vi "form voltage alarm string.old.vi"(0 "Xmon":dbl[][](array[numeric]), 1 "Xset":dbl[][](array[numeric]), 2 "Timestamps":dbl[][](array[numeric]), 3 "Alarm Tolerance (frac)":dbl=0.2 format="%#_13g", 4 "Warning Tolerance (frac)":dbl=0.1 format="%#_13g", 5 "error in":errorcluster, 6 "Alarm:T Warning:F":bool, 8 "Current:T Voltage:F":bool, 12 "Start index":i32) -> (14 "Error Status String":string, 15 "All channels in error":string, 17 "Error Array":string[][](array[string]), 19 "Error Out":errorcluster)   [LabVIEW 2015]
uses:
  CAEN globals.vi
  <userlib>/_OpenG.lib/array/array.llb/Search 1D Array (Boolean)__ogtk.vi
  <userlib>/_OpenG.lib/array/array.llb/Index 1D Array Elements (I32)__ogtk.vi
  <userlib>/_OpenG.lib/array/array.llb/Index 1D Array Elements (Boolean)__ogtk.vi
  <userlib>/_OpenG.lib/array/array.llb/Index 1D Array Elements (String)__ogtk.vi
  <userlib>/_OpenG.lib/array/array.llb/Index 1D Array Elements (DBL)__ogtk.vi
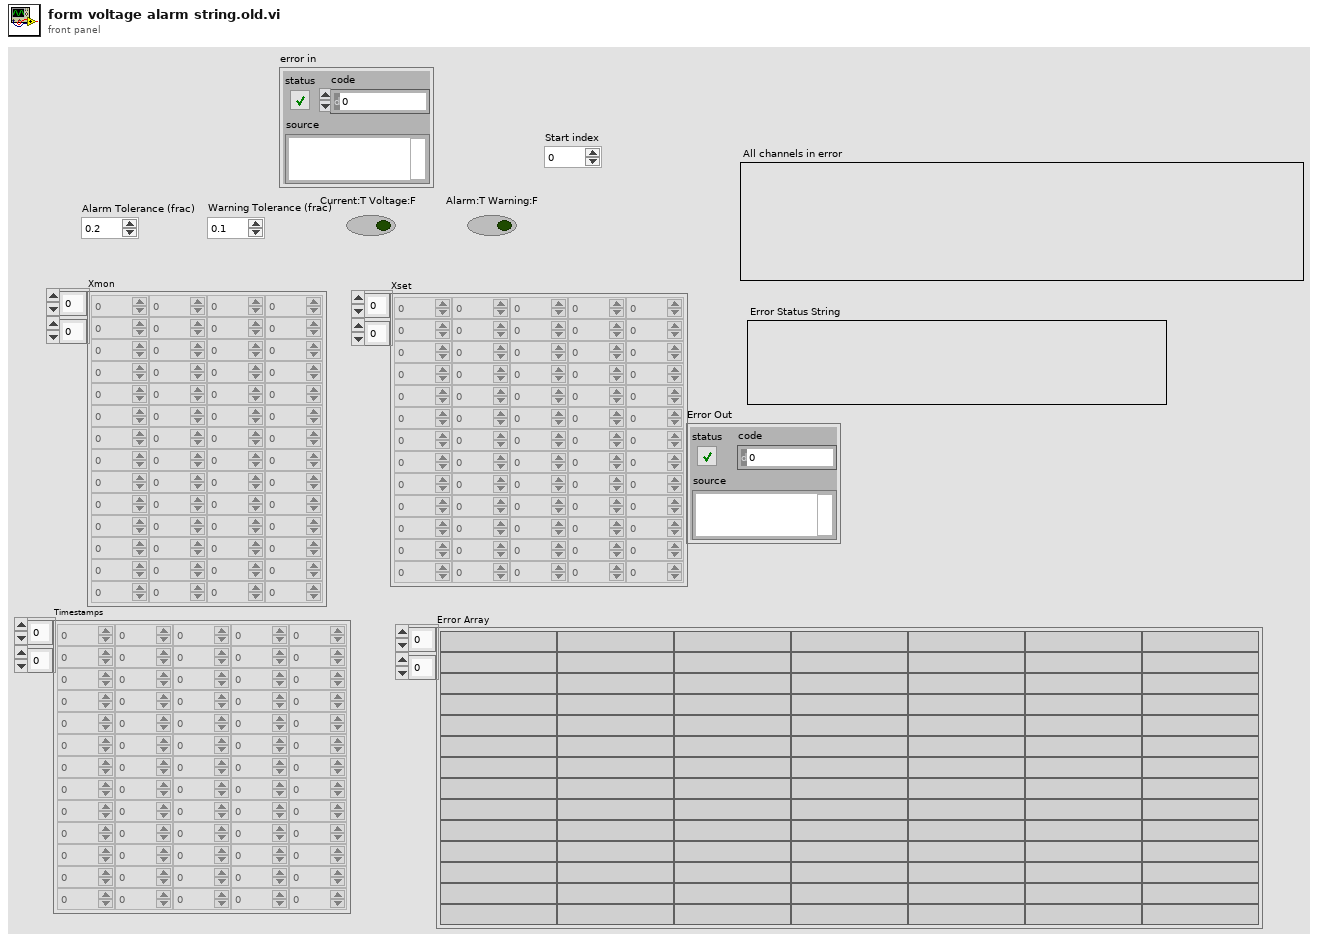
[diagram p1: front panel]
types:
  T1 = cluster{"Slot num":i32, "Indices of Elements":i32[]}[]
  T2 = cluster{"Channel Name":string, "Crate":i32, "Card Type":string, "Card":i32, "Channel":i32, "Status Icon":picture, "Vmon (V)":dbl, "Vset (V)":dbl, "Imon (A)":dbl, "Iset (A)":dbl, "Timestamp":string, "ON/OFF":bool, "Status":string, "Vswmax (V)":dbl}[]
  T3 = cluster{"Channel Name":string, "Crate":i32, "Card Type":string, "Card":i32, "Channel":i32, "Status Icon":picture, "Vmon (V)":dbl, "Vset (V)":dbl, "Imon (A)":dbl, "Iset (A)":dbl, "Timestamp":string, "ON/OFF":bool, "Status":string, "Vswmax (V)":dbl}
  T4 = cluster{"Numeric":i32, "Indices of Elements":i32[]}
  T5 = cluster{"Numeric":i32, "Indices of Elements":i32[]}[]
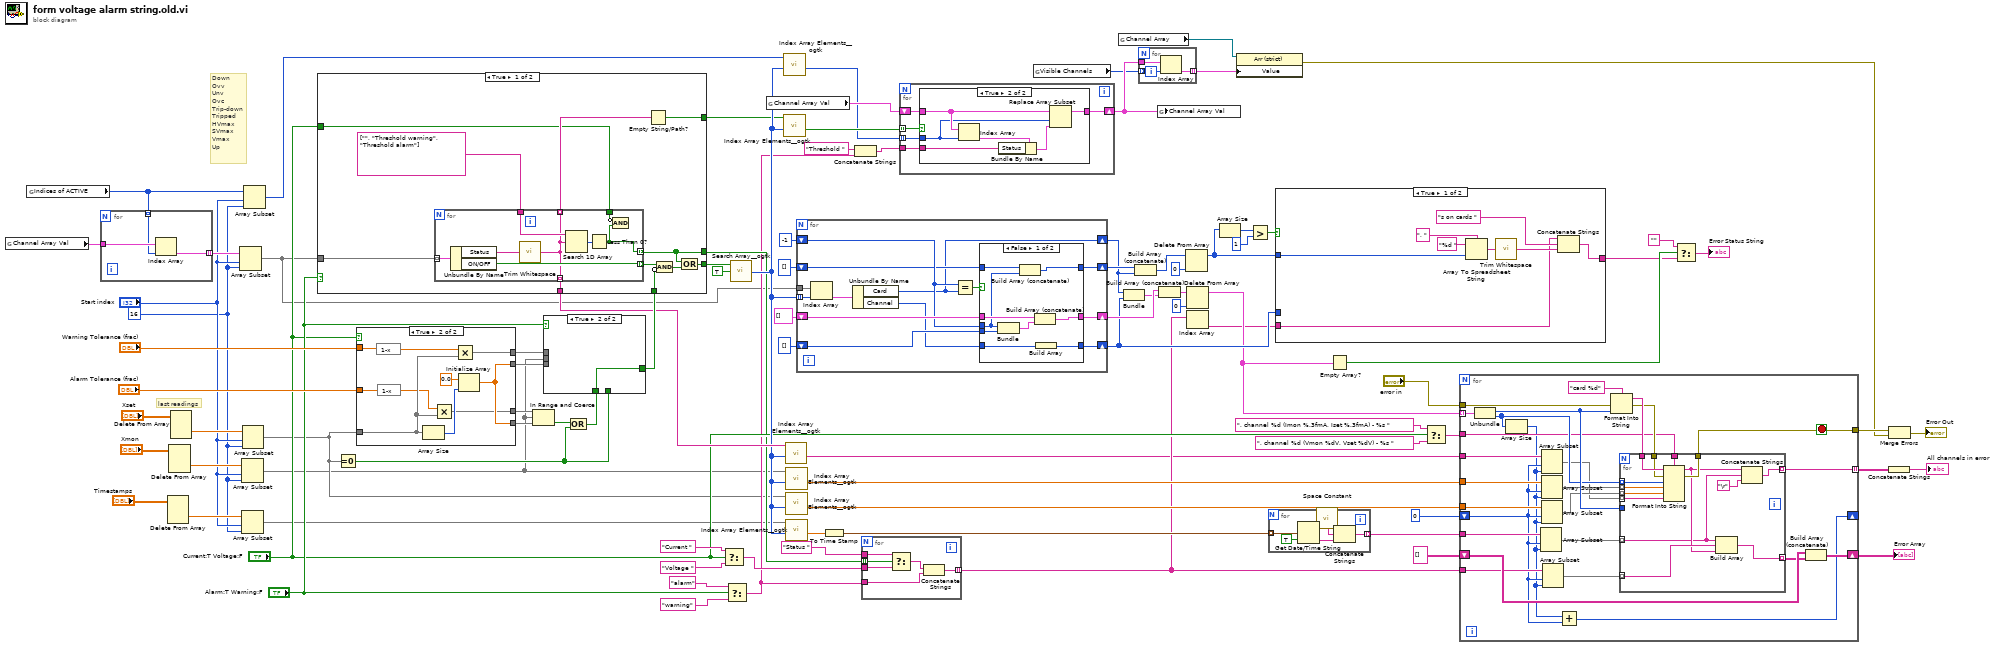
[diagram p0: block diagram]
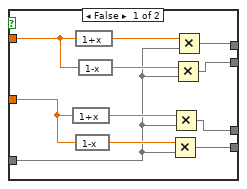
[diagram p3: hidden frame]
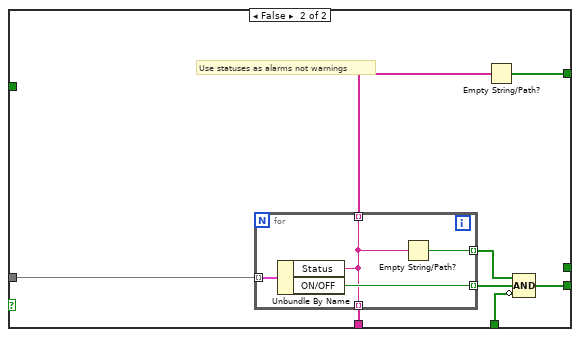
[diagram p4: hidden frame]
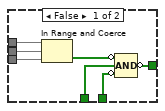
[diagram p5: hidden frame]
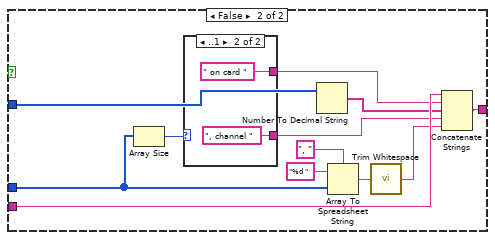
[diagram p6: hidden frame]
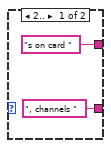
[diagram p7: hidden frame]
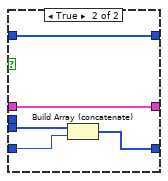
[diagram p8: hidden frame]
diagram:
  w2 = 16 ("Length")
  # "Down\nOvv\nUnv\nOvc\nTrip-down\nTripped\nHVmax\nSVmax\nVmax\nUp"
  # "last readings"
  n1 = global read "CAEN globals.vi" "Channel Array Val"() -> (w39:T2)
  n2 = global read "CAEN globals.vi" "Indices of ACTIVE"() -> (w5:i32[])
  n3 = for {
    tunnel: w39 -> [w95]
    tunnel: [w94] -> w6 mode=indexing
    tunnel: w5 -> [w93] mode=indexing
    n4 = Index Array(array=w95, index=w93) -> (element=w94:T3)
  }
  n5 = Delete From Array(array="Timestamps") -> (deleted portion=w9:dbl[])  [unwired: 3 in, 1 out]
  n6 = Delete From Array(array="Xmon") -> (deleted portion=w11:dbl[])  [unwired: 3 in, 1 out]
  n7 = Delete From Array(array="Xset") -> (deleted portion=w13:dbl[])  [unwired: 3 in, 1 out]
  n8 = Array Subset(array=w6, index="Start index", length=w2) -> (w7:T2)
  n9 = Array Subset(array=w11, index="Start index", length=w2) -> (w10:dbl[])
  n10 = Array Subset(array=w9, index="Start index", length=w2) -> (w8:dbl[])
  n11 = Array Subset(array=w13, index="Start index", length=w2) -> (w12:dbl[])
  n12 = Array Subset(array=w5, index="Start index", length=w2) -> (w4:i32[])
  n13 = Equal To 0?(x=w12) -> (x = 0?=w46:bool[])
  n14 = case shown="True" "Current:T Voltage:F" {
    tunnel: [w98 w114] -> w63
    tunnel: [w99 w109] -> w62
    tunnel: [w104 w111] -> w45
    tunnel: [w102 w114] -> w44
    tunnel: "Warning Tolerance (frac)" -> [w106 w112]
    tunnel: "Alarm Tolerance (frac)" -> [w97 w110]
    tunnel: w12 -> [w96 w113]
    frame False {
      n15 = expression code="1+x"(w97) -> (w100:dbl)
      n16 = expression code="1+x"(w106) -> (w105:dbl)
      n17 = expression code="1-x"(w97) -> (w101:dbl)
      n18 = expression code="1-x"(w106) -> (w103:dbl)
      n19 = Multiply(x=w101, y=w96) -> (x*y=w98:dbl[])
      n20 = Multiply(x=w100, y=w96) -> (x*y=w99:dbl[])
      n21 = Multiply(x=w103, y=w96) -> (x*y=w102:dbl[])
      n22 = Multiply(x=w105, y=w96) -> (x*y=w104:dbl[])
    }
    frame True {
      n23 = expression code="1-x"(w112) -> (w108:dbl)
      n24 = expression code="1-x"(w110) -> (w107:dbl)
      n25 = Array Size(array=w113) -> (size(s)=w116:i32)
      n26 = Multiply(x=w107, y=w113) -> (x*y=w109:dbl[])
      n27 = Multiply(x=w108, y=w113) -> (x*y=w111:dbl[])
      n28 = Initialize Array(0.0 ("element"), w116) -> (w114:dbl[])
    }
  }
  n29 = In Range and Coerce(upper limit=w62, x=w10, lower limit=w63) -> (In Range?=w34:bool[])  [unwired: 1 out]
  n30 = Compound Arithmetic op=OR(w34, w46) -> (w33:bool[])
  n31 = case shown="True" "Alarm:T Warning:F" {
    tunnel: w10 -> [w123 _]
    tunnel: w33 -> [w121 w124]
    tunnel: [w120 w124] -> w49
    tunnel: w46 -> [w119 _]
    tunnel: w45 -> [w118 _]
    tunnel: w44 -> [w117 _]
    frame False {
      n32 = In Range and Coerce(upper limit=w118, x=w123, lower limit=w117) -> (In Range?=w122:bool[])  [unwired: 1 out]
      n33 = Compound Arithmetic op=AND(invert w122, w121, invert w119) -> (invert w120:bool[])
    }
    frame True {
    }
  }
  n34 = case shown="True" "Alarm:T Warning:F" {
    tunnel: [w131 w148] -> w48
    tunnel: w49 -> [w129 w150]
    tunnel: [w135 w151] -> w47
    tunnel: [w134 w145] -> w20
    tunnel: w7 -> [w132 w144]
    tunnel: "Current:T Voltage:F" -> [w126 _]
    tunnel: [w125 _] -> w19
    frame True {
      n35 = for {
        tunnel: w132 -> [w143] mode=indexing
        tunnel: [w140] -> w130 mode=indexing
        tunnel: [w136] -> w125 mode=indexing
        tunnel: string[] ["", "Threshold warning", "Threshold alarm"] ("items to filter") -> [w141]
        tunnel: [w137] -> w135 mode=indexing
        tunnel: [w137] -> w133 mode=indexing
        tunnel: w126 -> [w139]
        n36 = Unbundle By Name(w143) -> ("Status"=w138:string, "ON/OFF"=w140:bool)
        n37 = call <vilib>:"Trim Whitespace.vi"("string"=w138) -> ("trimmed string"=w137:string)  [unwired: 1 in]
        n38 = Search 1D Array(1D array=w141, element=w137) -> (index of element=w142:i32)  [unwired: 1 in]
        n39 = Less Than 0?(x=w142) -> (x < 0?=w136:bool)
        n40 = Compound Arithmetic op=AND(invert w139, w136) -> ()  [unwired: 1 out]
      }
      n41 = Empty String/Path?(string/path=w133) -> (empty?=w134:bool[])
      n42 = Compound Arithmetic op=AND(w130, invert w129) -> (w128:bool[])
      n43 = Compound Arithmetic op=OR(w125, w128) -> (w131:bool[])
    }
    frame False {
      # "Use statuses as alarms not warnings"
      n44 = for {
        tunnel: w144 -> [w155] mode=indexing
        tunnel: [w152] -> w147 mode=indexing
        tunnel: [w153] -> w151 mode=indexing
        tunnel: [w154] -> w149 mode=indexing
        tunnel: [w153] -> w146 mode=indexing
        n45 = Unbundle By Name(w155) -> ("Status"=w153:string, "ON/OFF"=w154:bool)
        n46 = Empty String/Path?(string/path=w153) -> (empty?=w152:bool)
      }
      n47 = Empty String/Path?(string/path=w146) -> (empty?=w145:bool[])
      n48 = Compound Arithmetic op=AND(w147, w149, invert w150) -> (w148:bool[])
    }
  }
  n49 = Select(t="Current " ("Card type"), s="Current:T Voltage:F", f="Voltage " ("Card type")) -> (s? t:f=w17:string)
  n50 = Select(t="alarm" ("Card type"), s="Alarm:T Warning:F", f="warning" ("Card type")) -> (s? t:f=w16:string)
  n51 = call-poly <userlib>:"Search Array__ogtk.vi"("Array"=w48, "Element Data"=TRUE) -> ("Indices of Elements"=w40:i32[])  [unwired: 7 in]
  n52 = global read "CAEN globals.vi" "Channel Array Val"() -> (w29:T2)
  n53 = call-poly <userlib>:"Index Array Elements__ogtk.vi"("indices"=w40, "array"=w4) -> ("elements"=w24:i32[])  [unwired: 9 in]
  n54 = call-poly <userlib>:"Index Array Elements__ogtk.vi"("indices"=w40, "array"=w20) -> ("elements"=w32:bool[])  [unwired: 9 in]
  n55 = call-poly <userlib>:"Index Array Elements__ogtk.vi"("indices"=w40, "array"=w47) -> ("elements"=w1:string[])  [unwired: 9 in]
  n56 = call-poly <userlib>:"Index Array Elements__ogtk.vi"("indices"=w40, "array"=w10) -> ("elements"=w60:dbl[])  [unwired: 9 in]
  n57 = call-poly <userlib>:"Index Array Elements__ogtk.vi"("indices"=w40, "array"=w12) -> ("elements"=w59:dbl[])  [unwired: 9 in]
  n58 = call-poly <userlib>:"Index Array Elements__ogtk.vi"("indices"=w40, "array"=w8) -> ("elements"=w50:dbl[])  [unwired: 9 in]
  n59 = for {
    tunnel: w40 -> [w160] mode=indexing
    shift-right: [w157] -> w57
    shift-left: -1 ("Numeric") -> [w163]
    shift-right: [w167] -> w72
    shift-left: i32[] [] ("Indices of Elements") -> [w168]
    shift-right: [w165] -> w76
    shift-left: T1 [] -> [w164]
    shift-right: [w161] -> w58
    shift-left: i32[] [] ("Indices of Elements") -> [w162]
    tunnel: w7 -> [w159]
    n60 = Index Array(array=w159, index=w160) -> (element=w158:T3)
    n61 = Unbundle By Name(w158) -> ("Card"=w157:i32, "Channel"=w156:i32)
    n62 = Equal?(x=w163, y=w157) -> (x = y?=w166:bool)
    n63 = case shown="False" w166 {
      tunnel: w168 -> [w175 w182]
      tunnel: w156 -> [w177 w181]
      tunnel: [w176 w180] -> w167
      tunnel: [w173 w179] -> w165
      tunnel: w164 -> [w172 w179]
      tunnel: w163 -> [w170 _]
      tunnel: w162 -> [w171 w178]
      tunnel: [w169 w178] -> w161
      frame False {
        n64 = Bundle("Numeric"=w170, "Indices of Elements"=w175) -> (w174:T4)  [unwired: 1 in]
        n65 = Build Array (concatenate)(w171, w170) -> (w169:i32[])
        n66 = Build Array (concatenate)(w172, w174) -> (w173:T5)
        n67 = Build Array(w177) -> (w176:i32[])
      }
      frame True {
        n68 = Build Array (concatenate)(w182, w181) -> (w180:i32[])
      }
    }
  }
  n69 = To Time Stamp(1:w50) -> (0:w23:timestamp[])
  n70 = Concatenate Strings("Threshold " ("string"), w16) -> (w31:string)
  n71 = for {
    tunnel: w19 -> [w188] mode=indexing
    tunnel: "Status " ("Card type") -> [w187]
    tunnel: w17 -> [w186]
    tunnel: w16 -> [w184]
    tunnel: [w183] -> w15 mode=indexing
    n72 = Select(t=w187, s=w188, f=w186) -> (s? t:f=w185:string)
    n73 = Concatenate Strings(w185, w184) -> (w183:string)
  }
  n74 = for {
    shift-right: [w190] -> w28
    shift-left: w29 -> [w193]
    tunnel: w32 -> [w192] mode=indexing
    tunnel: w24 -> [w191] mode=indexing
    tunnel: w31 -> [w189]
    n75 = case shown="True" w192 {
      tunnel: w193 -> [w194 w199]
      tunnel: w191 -> [_ w198]
      tunnel: [w194 w200] -> w190
      tunnel: w189 -> [_ w195]
      frame False {
      }
      frame True {
        n76 = Index Array(array=w199, index=w198) -> (element=w197:T3)
        n77 = Bundle By Name(cluster=w197, "Status"=w195) -> (w196:T3)
        n78 = Replace Array Subset(array=w199, new element=w196, index=w198) -> (w200:T2)
      }
    }
  }
  n79 = global read "CAEN globals.vi" "Visible Channels"() -> (w27:i32[])
  n80 = global read "CAEN globals.vi" "Channel Array"() -> (w26:refnum<vi>)
  n81 = Bundle("Numeric"=w57, "Indices of Elements"=w72) -> (w75:T4)  [unwired: 1 in]
  n82 = Build Array (concatenate)(w58, w57) -> (w56:i32[])
  n83 = for {
    tunnel: w28 -> [w203]
    tunnel: w27 -> [w202] mode=indexing
    tunnel: [w201] -> w25 mode=indexing
    n84 = Index Array(array=w203, index=w202) -> (element=w201:T3)
  }
  n85 = global write "CAEN globals.vi" "Channel Array Val"(w28) -> ()
  n86 = Build Array (concatenate)(w76, w75) -> (w74:T5)
  n87 = Delete From Array(array=w56, index=0) -> (array with subset deleted=w55:i32[])  [unwired: 1 in, 1 out]
  n88 = Delete From Array(array=w74, index=0) -> (array with subset deleted=w71:T5)  [unwired: 1 in, 1 out]
  n89 = Index Array(array=w15) -> (element=w14:string)  [unwired: 1 in]
  n90 = Array Size(array=w55) -> (size(s)=w89:i32)
  n91 = property class="Arr (strict)"(reference=w26, "Value"=w25) -> (error out=w36:errorcluster)  [unwired: 1 in, 1 out]
  n92 = Greater?(x=w89, y=1) -> (0:w87:bool)
  n93 = for {
    tunnel: w23 -> [w205] mode=indexing
    tunnel: [w204] -> w22 mode=indexing
    n94 = Get Date/Time String(seconds (now)=w205, want seconds? (F)=TRUE) -> (date string=w208:string, time string=w206:string)  [unwired: 1 in]
    n95 = call <vilib>:"Space Constant.vi"() -> ("String"=w209:string)
    n96 = Concatenate Strings(w208, w209, w206) -> (w204:string)
  }
  n97 = case shown="True" w87 {
    tunnel: w55 -> [w211 w228]
    tunnel: [w215 w229] -> w53
    tunnel: w72 -> [_ w227]
    tunnel: w14 -> [w210 w226]
    frame True {
      n98 = Array To Spreadsheet String(delimiter (Tab)=", ", array=w211, 3:"%d " ("delimiter (Tab)")) -> (spreadsheet string=w213:string)
      n99 = call <vilib>:"Trim Whitespace.vi"("string"=w213) -> ("trimmed string"=w212:string)  [unwired: 1 in]
      n100 = Concatenate Strings(w210, "s on cards " ("Card type"), w212) -> (w215:string)
    }
    frame False {
      n101 = Array Size(array=w227) -> (size(s)=w220:i32)
      n102 = case shown="..1" w220 {
        tunnel: [", channels " ("Card type") ", channel " ("Card type")] -> w219
        tunnel: ["s on card " ("Card type") " on card " ("Card type")] -> w218
        frame 2.. {
        }
        frame ..1 {
        }
      }
      n103 = Number To Decimal String(number=w228) -> (decimal integer string=w222:string[])  [unwired: 1 in]
      n104 = Array To Spreadsheet String(delimiter (Tab)=", ", array=w227, 3:"%d " ("delimiter (Tab)")) -> (spreadsheet string=w224:string)
      n105 = call <vilib>:"Trim Whitespace.vi"("string"=w224) -> ("trimmed string"=w223:string)  [unwired: 1 in]
      n106 = Concatenate Strings(w226, w218, w222, w219, w223) -> (w229:string)
    }
  }
  n107 = Empty Array?(array=w71) -> (empty?=w92:bool)
  n108 = Select(t=", channel %d (Imon %.3fmA, Iset %.3fmA) - %s " ("delimiter (Tab)"), s="Current:T Voltage:F", f=", channel %d (Vmon %dV, Vset %dV) - %s " ("delimiter (Tab)")) -> (s? t:f=w51:string)
  n109 = for {
    tunnel: w60 -> [w250]
    tunnel: w59 -> [w248]
    tunnel: w71 -> [w254] mode=indexing
    tunnel: w51 -> [w238]
    tunnel: [w258] -> w84 mode=indexing
    shift-right: [w257] -> w81
    shift-left: string[][] [] -> [w256]
    tunnel: w15 -> [w236]
    shift-right: [w246] -> _
    shift-left: 0 -> [w235]
    tunnel: "error in" -> [w245]
    tunnel: [w243] -> w38
    tunnel: w22 -> [w240]
    tunnel: w1 -> [w242]
    stop <- w243 stop-if-true
    n110 = Unbundle(w254) -> ("Numeric"=w253:i32, "Indices of Elements"=w251:i32[])
    n111 = Array Size(array=w251) -> (size(s)=w234:i32)
    n112 = Array Subset(array=w240, index=w235, length=w234) -> (w239:string[])
    n113 = Array Subset(array=w242, index=w235, length=w234) -> (w241:string[])
    n114 = Array Subset(array=w250, index=w235, length=w234) -> (w249:dbl[])
    n115 = Array Subset(array=w248, index=w235, length=w234) -> (w247:dbl[])
    n116 = Array Subset(array=w236, index=w235, length=w234) -> (w237:string[])
    n117 = Add(x=w234, y=w235) -> (x+y=w246:i32)
    n118 = Format Into String(format string="card %d" ("Card type"), error in=w245, w253) -> (resulting string=w259:string, error out=w244:errorcluster)  [unwired: 1 in]
    n119 = for {
      tunnel: w251 -> [w267] mode=indexing
      tunnel: w249 -> [w270] mode=indexing
      tunnel: w247 -> [w269] mode=indexing
      tunnel: w238 -> [w273]
      tunnel: w259 -> [w272]
      tunnel: [w261] -> w258 mode=indexing
      tunnel: [w271] -> w243
      tunnel: w253 -> [_]
      tunnel: [w268] -> w255 mode=indexing
      tunnel: w237 -> [w264] mode=indexing
      tunnel: w244 -> [w266]
      tunnel: w239 -> [w260] mode=indexing
      tunnel: w241 -> [w265] mode=indexing
      n120 = Format Into String(format string=w273, initial string=w272, error in=w266, w267, w270, w269, w265) -> (resulting string=w263:string, error out=w271:errorcluster)
      n121 = Build Array(w260, w264, w263) -> (w268:string[])
      n122 = Concatenate Strings(w263, w260, "\r") -> (w261:string)
    }
    n123 = Build Array (concatenate)(w256, w255) -> (w257:string[][])
  }
  "Error Array" <- w81
  n124 = Select(t="", s=w92, f=w53) -> (s? t:f=→"Error Status String":string)
  n125 = Concatenate Strings(w84) -> (→"All channels in error":string)
  n126 = Merge Errors(w38, w36) -> (→"Error Out":errorcluster)
